vi "Read RemIO Module Page Property.vi"(8 "error in (no error)":errorcluster, 11 "Node Ptr In":T1 format="%.0x") -> (0 "error out":errorcluster, 2 "RemIO Module":refnum<class "RemIO Module.lvclass">, 3 "Node Ptr Out":T1 format="%.0x")   [LabVIEW 2019, in "Modules.lvlib" / "RemIO Module.lvclass"]
uses:
  RemIO Module.lvclass
  <vilib>/NI VeriStand/Custom Device API/Custom Device Item Ref.ctl
  RSI Module/Class Property Strings.vi
  <vilib>/NI VeriStand/Custom Device API/Get Item Property (String).vi
  <vilib>/NI VeriStand/Custom Device API/Custom Device API.lvlib
  RSI Module/RSI Module.lvclass
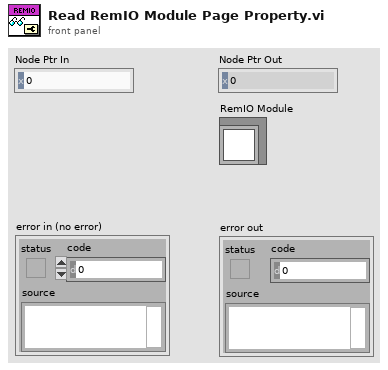
[diagram p1: front panel]
types:
  T1 = typedef "Custom Device API.lvlib/Custom Device Item Ref.ctl" = u64
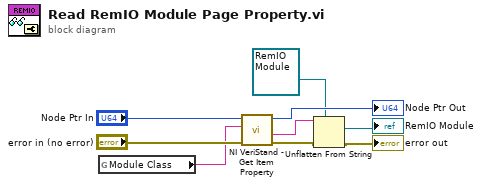
[diagram p0: block diagram]
diagram:
  n1 = global read "Class Property Strings.vi" "Module Class"() -> (w3:string)
  n2 = call-poly <vilib>:"NI VeriStand - Get Item Property.vi"("error in (no error)"="error in (no error)", "Property Name"=w3, "Item Ref in"="Node Ptr In") -> ("error out"=w5:errorcluster, "Value"=w4:string, "Item Ref out"=→"Node Ptr Out":T1)  [unwired: 5 in, 1 out]
  n3 = Unflatten From String(type=refnum<class "RemIO Module.lvclass"> refnum ("Modules.lvlib:RemIO Module.lvclass"), binary string=w4, error in (no error)=w5) -> (value=→"RemIO Module":refnum<class "RemIO Module.lvclass">, error out=→"error out":errorcluster)  [unwired: 2 in, 1 out]
